vi "Write.vi"(7 "Slave Address":u8, 8 "Error In":errorcluster, 10 "Data":u8[](array[numeric]), 11 "AD2 I2C In":refnum<class "AD2 I2C.lvclass">) -> (0 "Error Out":errorcluster, 3 "AD2 I2C Out":refnum<class "AD2 I2C.lvclass">)   [LabVIEW 2020, in "lv_i2c_ad2.lvlib" / "AD2 I2C.lvclass"]
uses:
  AD2 I2C.lvclass
  AD2 I2C.lvclass/AD2 I2C.ctl
  lv_waveforms_toolkit/lv_waveforms_toolkit.lvlib
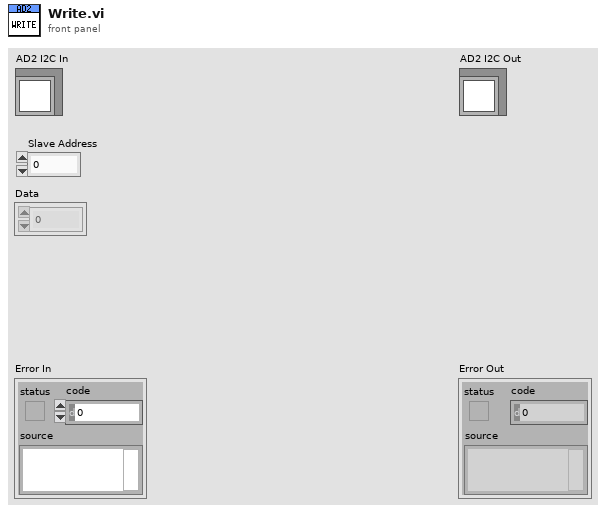
[diagram p1: front panel]
types:
  T1 = typedef "lv_waveforms_toolkit.lvlib/WFT Session.ctl" = cluster{"phdwf":i32, "Analog IO Configured":bool}
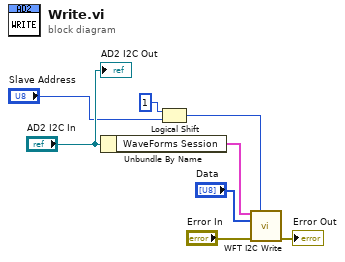
[diagram p0: block diagram]
diagram:
  n1 = Unbundle By Name("AD2 I2C In") -> ("WaveForms Session"=w5:T1)
  n2 = Logical Shift(y=i16 1, x="Slave Address") -> (x << y=w1:u8)
  n3 = call "WFT I2C Write.vi"("WaveForms Session In"=w5, "adr8Bits"=w1, "rgbTx"="Data", "Error In"="Error In") -> ("Error Out"=→"Error Out":errorcluster)  [unwired: 8 in, 3 out]
  "AD2 I2C Out" <- "AD2 I2C In"
